vi "Find Workspace.vi"(8 "Error In":errorcluster, 10 "Control In":T2={"I-O.lvclass"=refnum, "Motion.lvclass"=refnum, "Dispenser.lvclass"=refnum}, 11 "Workspace In":refnum<class "Current Position.lvclass">) -> (0 "Error Out":errorcluster, 1 "Workspace Out":T1, 2 "Control Out":T2, 3 "Workspace Out":refnum<class "Current Position.lvclass">)   [LabVIEW 2016, in "Current Position.lvclass"]
uses:
  Current Position.lvclass
  Controller/Controllers.ctl
  Controller/I-O/I-O.lvclass
  Controller/Motion/A3200/A3200.lvclass
  Controller/Dispenser/Dispenser.lvclass
  Controller/Motion/Motion.lvclass
  Workspace.ctl
  Controller/Controller.lvclass
  Fixture.lvclass
panel:
  in  "Workspace":T1
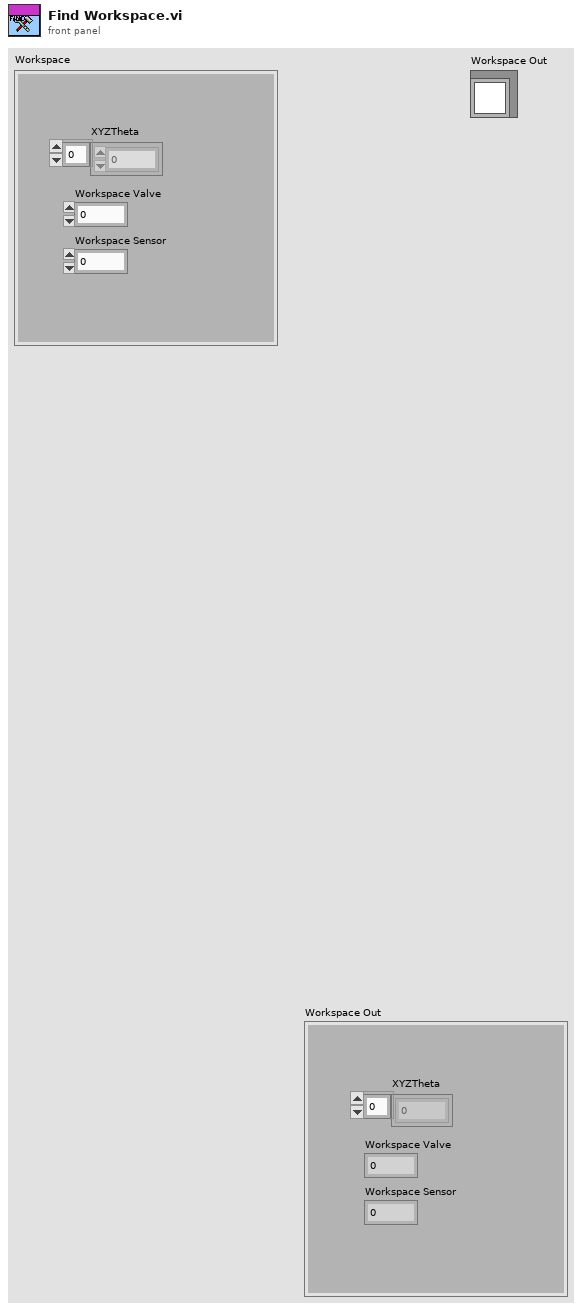
[diagram p1: front panel]
types:
  T1 = typedef "Fixture.lvclass/Workspace.ctl" = cluster{"XYZTheta":dbl[], "Workspace Valve":i32, "Workspace Sensor":i32}
  T2 = typedef "Controller.lvclass/Controllers.ctl" = cluster{"I-O.lvclass":refnum<class "I-O.lvclass">, "Motion.lvclass":refnum<class "Motion.lvclass">, "Dispenser.lvclass":refnum<class "Dispenser.lvclass">}
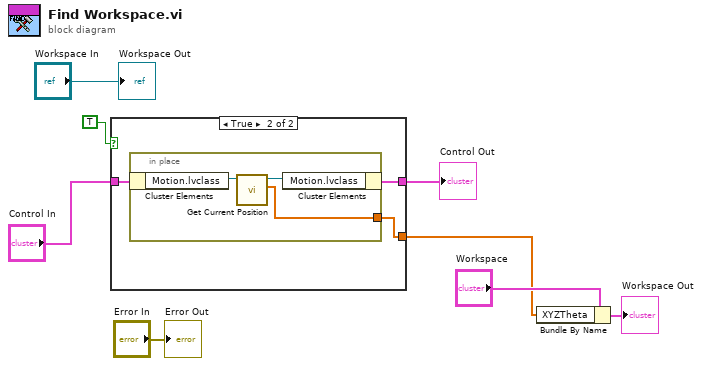
[diagram p0: block diagram]
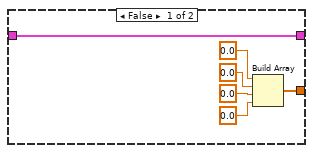
[diagram p2: hidden frame]
diagram:
  n1 = case shown="True" TRUE {
    tunnel: "Control In" -> [w14 w17]
    tunnel: [w14 w16] -> w7
    tunnel: [w13 w15] -> w5
    frame False {
      n2 = Build Array(0.0, 0.0, 0.0, 0.0) -> (w13:dbl[])
    }
    frame True {
      n3 = in-place {
        in-place-border: [w18] -> w15
        n4 = in-place-cluster #1(w17) -> ("Motion.lvclass"=w20:refnum<class "Motion.lvclass">)
        n5 = call-dynamic "Get Current Position.vi"("Motion in"=w20) -> ("XYZTheta Out"=w18:dbl[], "Motion out"=w19:refnum<class "Motion.lvclass">)  [unwired: 8 in, 1 out]
        n6 = in-place-cluster #1("Motion.lvclass"=w19) -> (w16:T2)
      }
    }
  }
  "Control Out" <- w7
  n7 = Bundle By Name(cluster="Workspace", "XYZTheta"=w5) -> (→"Workspace Out":T1)
  "Error Out" <- "Error In"
  "Workspace Out" <- "Workspace In"
